vi "Test Log No Warning Recorded Without Message.vi"(8 "error in (no error)":errorcluster, 11 "Test Case In":refnum<class "Logger Test.lvclass">) -> (0 "error out":errorcluster, 3 "Test Case Out":refnum<class "Logger Test.lvclass">)   [LabVIEW 2020, in "Logger Test.lvclass"]
uses:
  Logger Test.lvclass
  C:/Program Files (x86)/National Instruments/LabVIEW 2020/vi.lib/Asteme/LUnit/Test Case.lvclass
  Mock Process/Mock Process.lvclass
  C:/Users/anton/Documents/GitHub/Triarc-Framework/source/Framework/Process/Process.lvclass
  C:/Users/anton/Documents/GitHub/Triarc-Framework/source/Framework/Logging/Logging.lvclass
  Mock Log Handler/Mock Log Handler.lvclass
  <vilib>/Asteme/LUnit/Test Case.lvclass/Test Case.ctl
  <vilib>/Asteme/LUnit/LUnit Assertion Result.lvclass/LUnit Assertion Result.ctl
  <vilib>/Asteme/LUnit/Palette/Fail.vi
  <vilib>/Asteme/LUnit/Palette/Pass.vi
  <vilib>/Asteme/LUnit/Set Assertion Type.vi
  <vilib>/Asteme/LUnit/Add test result.vi
  <vilib>/Asteme/LUnit/LUnit Write Passed.vi
  <vilib>/Asteme/LUnit/LUnit Get Test Case.vi
  <vilib>/Asteme/LUnit/LUnit Write Message.vi
  <vilib>/Asteme/LUnit/LUnit Write Description.vi
  <vilib>/Asteme/LUnit/LUnit Write Assertion Type.vi
  <vilib>/Asteme/LUnit/Read Test Case Name.vi
  <vilib>/Asteme/LUnit/Assertion Result/LUnit Get Test Name.vi
  <vilib>/Asteme/LUnit/LUnit Assertion Result.lvclass
  Framework/Process/Process.lvclass
  Framework/Logging/Logging.lvclass
  <vilib>/Asteme/LUnit/Test Case.lvclass
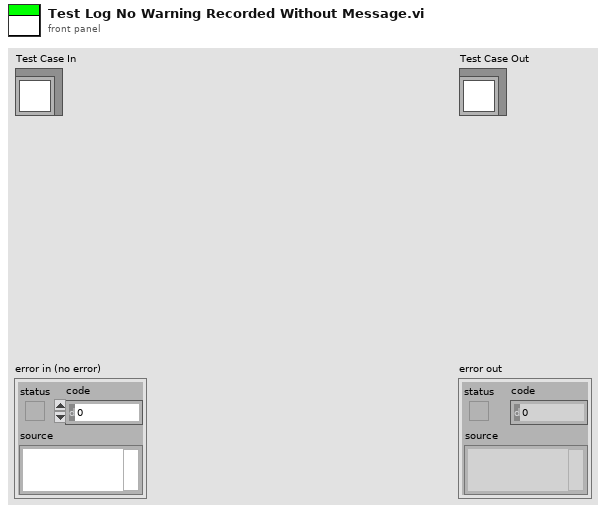
[diagram p1: front panel]
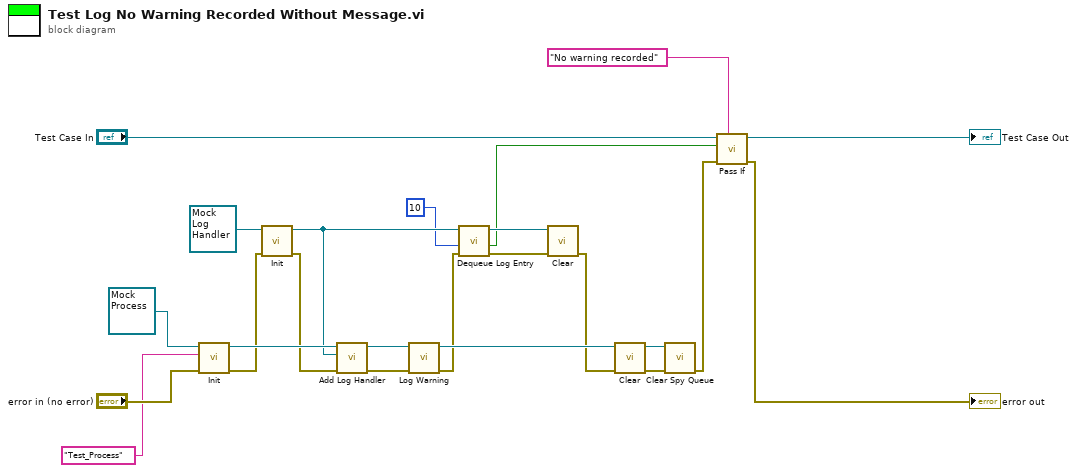
[diagram p0: block diagram]
diagram:
  n1 = call-dynamic "Init.vi"("error in (no error)"="error in (no error)", "Name"="Test_Process", "Mock Process In"=refnum<class "Mock Process.lvclass"> refnum) -> ("error out"=w14:errorcluster, "Mock Process Out"=w21:refnum<class "Mock Process.lvclass">)  [unwired: 7 in]
  n2 = call-dynamic "Init.vi"("error in (no error)"=w14, "Mock Log Handler In"=refnum<class "Mock Log Handler.lvclass"> refnum ("Mock Log Handler.lvclass")) -> ("error out"=w13:errorcluster, "Mock Log Handler Out"=w10:refnum<class "Mock Log Handler.lvclass">)  [unwired: 8 in]
  n3 = call "Add Log Handler.vi"("error in (no error)"=w13, "Log Handler"=w10, "Process In"=w21) -> ("error out"=w20:errorcluster, "Process Out"=w8:refnum<class "Mock Process.lvclass">)  [unwired: 7 in]
  n4 = call "Log Warning.vi"("error in (no error)"=w20, "Logging In"=w8) -> ("error out"=w6:errorcluster, "Logging Out"=w7:refnum<class "Mock Process.lvclass">)  [unwired: 8 in]
  n5 = call "Dequeue Log Entry.vi"("error in (no error)"=w6, "timeout in ms (-1)"=10, "Mock Log Handler in"=w10) -> ("error out"=w11:errorcluster, "timed out?"=w1:bool, "Mock Log Handler out"=w12:refnum<class "Mock Log Handler.lvclass">)  [unwired: 5 in, 1 out]
  n6 = call-dynamic "Clear.vi"("error in (no error)"=w11, "Mock Log Handler In"=w12) -> ("error out"=w5:errorcluster)  [unwired: 8 in, 1 out]
  n7 = call-dynamic "Clear.vi"("error in (no error)"=w5, "Mock Process In"=w7) -> ("error out"=w18:errorcluster, "Mock Process Out"=w19:refnum<class "Mock Process.lvclass">)  [unwired: 8 in]
  n8 = call-dynamic "Clear Spy Queue.vi"("error in (no error)"=w18, "Mock Process In"=w19) -> ("error out"=w3:errorcluster)  [unwired: 8 in, 1 out]
  n9 = call <vilib>:"Pass If.vi"("Description"="No warning recorded", "error in (no error)"=w3, "Pass?"=w1, "Test Case In"="Test Case In") -> ("error out"=→"error out":errorcluster, "Test Case Out"=→"Test Case Out":refnum<class "Logger Test.lvclass">)  [unwired: 6 in]
